vi "Set Sub Object.vi"(8 "error in":errorcluster, 9 "Sub Object":refnum<class "Sub Object.lvclass">, 10 "Sub Index":u8, 11 "Obj Entry in":refnum<class "Object Entry.lvclass">) -> (0 "error out":errorcluster, 3 "Obj Entry out":refnum<class "Object Entry.lvclass">)   [LabVIEW 2020, in "CANopen.lvlib" / "Object Entry.lvclass"]
doc: "Sets the Sub Object associated with the specified sub index. If the specified sub index is not found it creates a new Sub Object with the specified sub index."
uses:
  Object Entry.lvclass
  Sub Object/Sub Object.lvclass
  Object Entry.lvclass/Object Entry.ctl
  Sub Objects Dictionary/Sub Objects Dictionary.lvclass
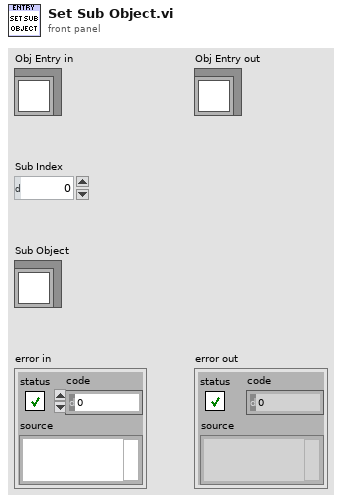
[diagram p1: front panel]
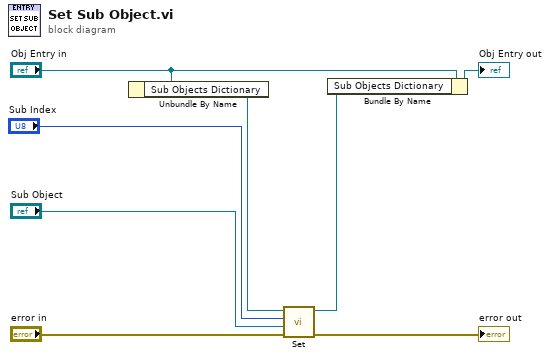
[diagram p0: block diagram]
diagram:
  n1 = Unbundle By Name("Obj Entry in") -> ("Sub Objects Dictionary"=w4:refnum<class "Sub Objects Dictionary.lvclass">)
  n2 = call "Set.vi"("error in"="error in", "Sub Object"="Sub Object", "Sub Index"="Sub Index", "Sub Objects Dictionary in"=w4) -> ("error out"=→"error out":errorcluster, "Sub Objects Dictionary out"=w3:refnum<class "Sub Objects Dictionary.lvclass">)  [unwired: 6 in]
  n3 = Bundle By Name(cluster="Obj Entry in", "Sub Objects Dictionary"=w3) -> (→"Obj Entry out":refnum<class "Object Entry.lvclass">)
